vi "ConfigureDlg.vi"(8 "error in (no error)":errorcluster, 11 "NiPxi6682 in":refnum<class "NiPxi6682.lvclass">) -> (0 "error out":errorcluster, 2 "Changed?":bool, 3 "NiPxi6682 out":refnum<class "NiPxi6682.lvclass">)   [LabVIEW 2014, in "SyncPlugins.lvlib" / "NiPxi6682.lvclass"]
uses:
  NiPxi6682.lvclass
  NiPxi6682.lvclass/NiPxi6682.ctl
  <userlib>/NIST/BaseClasses/BasePlugin_class/BasePlugin.lvclass/BasePlugin.ctl
  Accessors/Write 1PPS.vi
  Accessors/Write PgmPPS.vi
  Accessors/Write PgmPPSFreq.vi
  Accessors/Write DdsFreq.vi
  <userlib>/NIST/BaseClasses/BasePlugin_class/Accessors/Read PluginIniFilePath.vi
  Accessors/Read 1PPS.vi
  Accessors/Read PgmPPS.vi
  Accessors/Read PgmPPSFreq.vi
  Accessors/Read DdsFreq.vi
  <vilib>/Utility/config.llb/NI_LVConfig.lvlib
panel:
  in  "DDSFreq":dbl=100.0 caption="Backplane Clock Freq" format="%#.2p"
  in  "btnCancel":bool
  in  "btnDone":bool
  in  "Programmable Out Port":string
  in  "PgmPPSFreq":dbl=100.0 caption="Programable Out Freq"
  in  "PPS Out Port":string
  in  "Timing Card Handle":string
  in  "Clock Card Handle":string
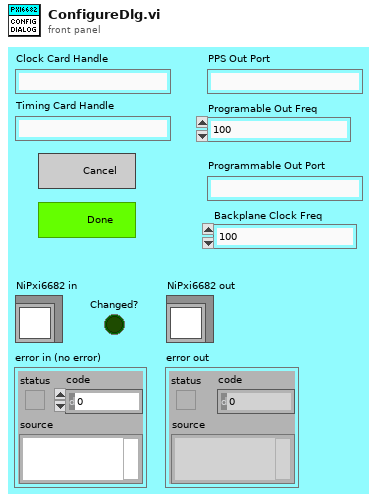
[diagram p1: front panel]
types:
  T1 = enum32{"Invalid", "Default", "Floating", "Floating/Auto-Hide", "Modal"}
  T2 = typedef "NI_LVConfig.lvlib/Config Data RefNum.ctl" = refnum<k1>
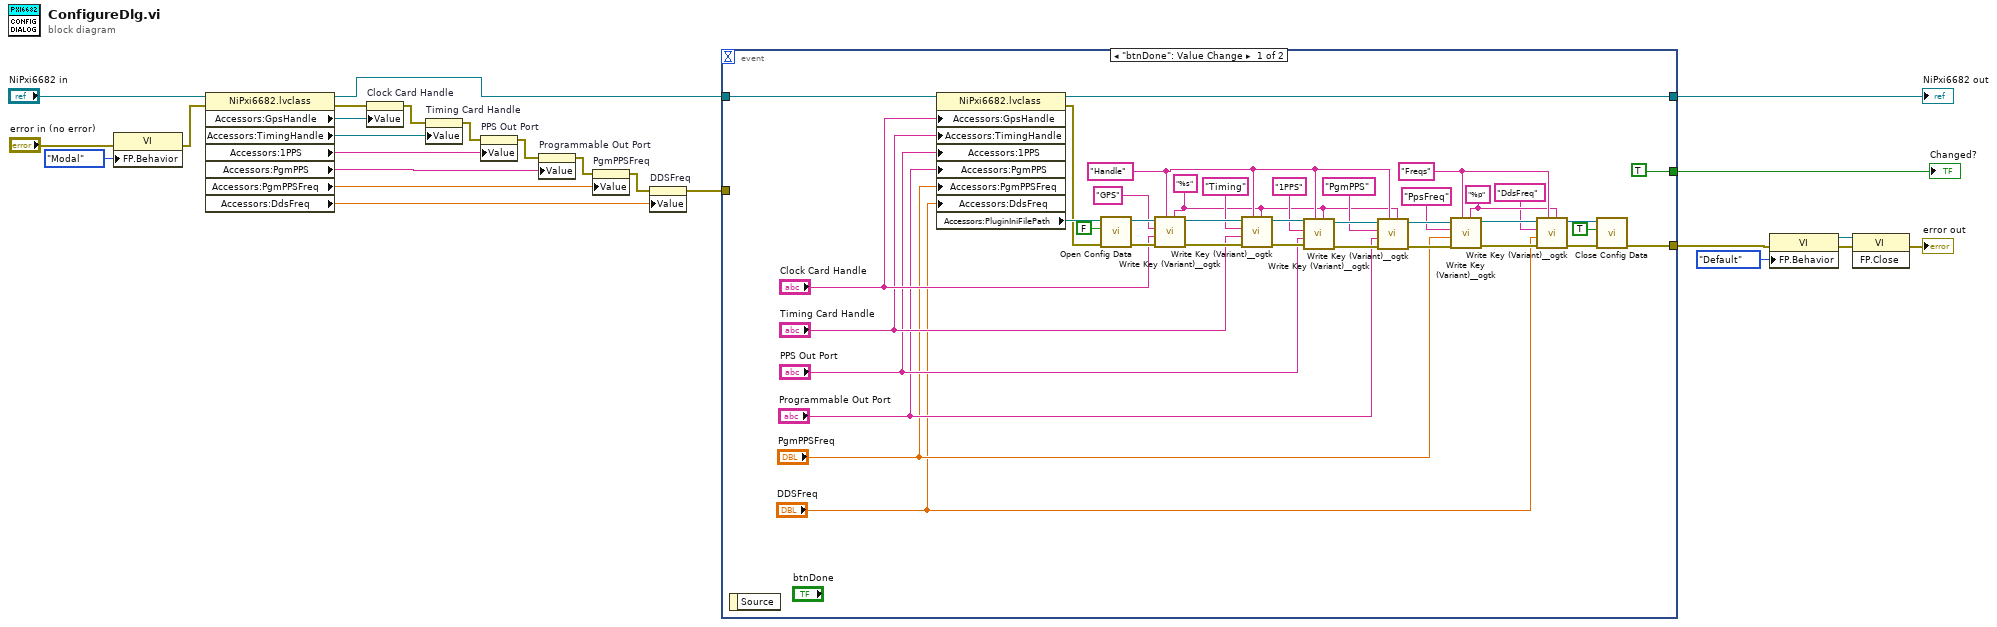
[diagram p0: block diagram]
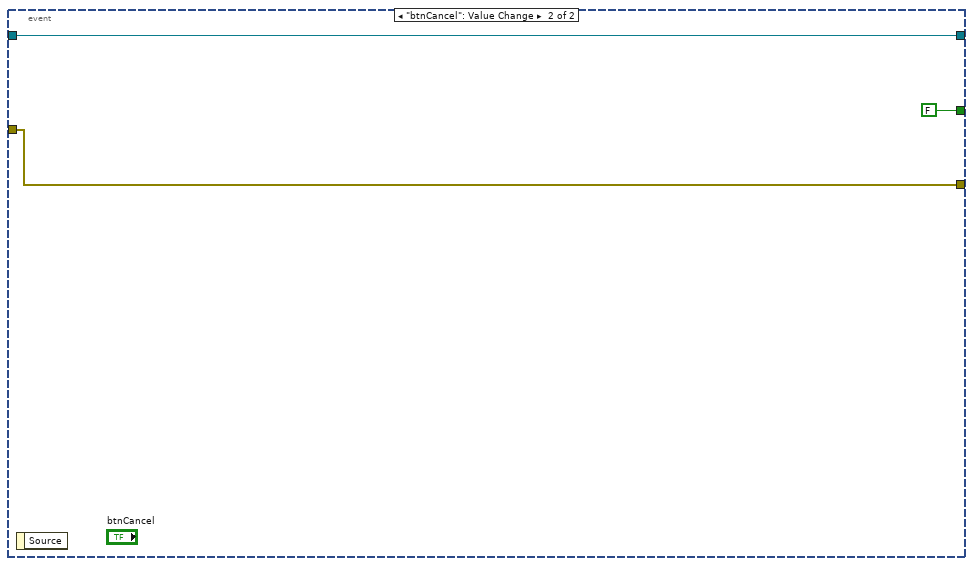
[diagram p2: hidden frame]
diagram:
  n1 = property class="VI"(error in="error in (no error)", "FP.Behavior"=T1."Modal" ("Front Panel Window:Behavior")) -> (error out=w22:errorcluster)  [unwired: 1 in, 1 out]
  n2 = property class="NiPxi6682.lvclass"(reference="NiPxi6682 in", error in=w22) -> (reference out=w7:refnum<class "NiPxi6682.lvclass">, error out=w17:errorcluster, "Accessors:GpsHandle"=w16:refnum<k15>, "Accessors:TimingHandle"=w15:refnum<k15>, "Accessors:1PPS"=w13:tag, "Accessors:PgmPPS"=w10:tag, "Accessors:PgmPPSFreq"=w9:dbl, "Accessors:DdsFreq"=w6:dbl)
  n3 = property on="Clock Card Handle" class="Str"(error in=w17, "Value"=w16) -> (error out=w14:errorcluster)  [unwired: 1 in, 1 out]
  n4 = property on="Timing Card Handle" class="Str"(error in=w14, "Value"=w15) -> (error out=w12:errorcluster)  [unwired: 1 in, 1 out]
  n5 = property on="PPS Out Port" class="Str"(error in=w12, "Value"=w13) -> (error out=w11:errorcluster)  [unwired: 1 in, 1 out]
  n6 = property on="Programmable Out Port" class="Str"(error in=w11, "Value"=w10) -> (error out=w8:errorcluster)  [unwired: 1 in, 1 out]
  n7 = property on="PgmPPSFreq" class="DigNum (strict)"(error in=w8, "Value"=w9) -> (error out=w5:errorcluster)  [unwired: 1 in, 1 out]
  n8 = property on="DDSFreq" class="DigNum (strict)"(error in=w5, "Value"=w6) -> (error out=w4:errorcluster)  [unwired: 1 in, 1 out]
  n9 = event shown="[0] \"btnDone\": Value Change" {
    selector: _ -> [_ _]
    dyn-events: _ -> [_ _]
    timeout: _ -> [_ _]
    tunnel: w7 -> [w63 w65]
    tunnel: w4 -> [_ w66]
    tunnel: [w28 w66] -> w3
    tunnel: [w27 w65] -> w2
    tunnel: [TRUE FALSE] -> w1
    event "btnDone": Value Change {
      w36 = "%p" ("float number format")
      w37 = "Freqs"
      w43 = "%s" ("float number format")
      w44 = "Handle"
      n10 = event-data() -> ()  [unwired: 1 in, 1 out]
      n11 = property class="NiPxi6682.lvclass"(reference=w63, "Accessors:GpsHandle"="Clock Card Handle", "Accessors:TimingHandle"="Timing Card Handle", "Accessors:1PPS"="PPS Out Port", "Accessors:PgmPPS"="Programmable Out Port", "Accessors:PgmPPSFreq"="PgmPPSFreq", "Accessors:DdsFreq"="DDSFreq") -> (reference out=w27:refnum<class "NiPxi6682.lvclass">, error out=w61:errorcluster, "Accessors:PluginIniFilePath"=w62:path)  [unwired: 1 in]
      n12 = call <vilib>:"Open Config Data.vi"("error in (no error)"=w61, "create file if necessary (T)"=FALSE, "configuration file path"=w62) -> ("error out"=w59:errorcluster, "refnum"=w58:T2)  [unwired: 6 in, 1 out]
      n13 = call <userlib>:"Write Key (Variant)__ogtk.vi"("float number format"=w43, "section"=w44, "error in (no error)"=w59, "key-value"="Clock Card Handle", "key (optional)"="GPS", "refnum"=w58) -> ("error out"=w56:errorcluster, "refnum out"=w55:T2)  [unwired: 4 in]
      n14 = call <userlib>:"Write Key (Variant)__ogtk.vi"("float number format"=w43, "section"=w44, "error in (no error)"=w56, "key-value"="Timing Card Handle", "key (optional)"="Timing", "refnum"=w55) -> ("error out"=w51:errorcluster, "refnum out"=w50:T2)  [unwired: 4 in]
      n15 = call <userlib>:"Write Key (Variant)__ogtk.vi"("float number format"=w43, "section"=w44, "error in (no error)"=w51, "key-value"="PPS Out Port", "key (optional)"="1PPS", "refnum"=w50) -> ("error out"=w47:errorcluster, "refnum out"=w46:T2)  [unwired: 4 in]
      n16 = call <userlib>:"Write Key (Variant)__ogtk.vi"("float number format"=w43, "section"=w44, "error in (no error)"=w47, "key-value"="Programmable Out Port", "key (optional)"="PgmPPS", "refnum"=w46) -> ("error out"=w41:errorcluster, "refnum out"=w40:T2)  [unwired: 4 in]
      n17 = call <userlib>:"Write Key (Variant)__ogtk.vi"("float number format"=w36, "section"=w37, "error in (no error)"=w41, "key-value"="PgmPPSFreq", "key (optional)"="PpsFreq", "refnum"=w40) -> ("error out"=w39:errorcluster, "refnum out"=w38:T2)  [unwired: 4 in]
      n18 = call <userlib>:"Write Key (Variant)__ogtk.vi"("float number format"=w36, "section"=w37, "error in (no error)"=w39, "key-value"="DDSFreq", "key (optional)"="DdsFreq", "refnum"=w38) -> ("error out"=w31:errorcluster, "refnum out"=w30:T2)  [unwired: 4 in]
      n19 = call <vilib>:"Close Config Data.vi"("error in (no error)"=w31, "write file if changed (T)"=TRUE, "refnum"=w30) -> ("error out"=w28:errorcluster)  [unwired: 7 in, 1 out]
    }
    event "btnCancel": Value Change {
      n20 = event-data() -> ()  [unwired: 1 in, 1 out]
    }
  }
  "NiPxi6682 out" <- w2
  "Changed?" <- w1
  n21 = property class="VI"(error in=w3, "FP.Behavior"=T1."Default" ("Front Panel Window:Behavior")) -> (reference out=w21:refnum<vi>, error out=w20:errorcluster)  [unwired: 1 in]
  n22 = invoke class="VI" method="FP.Close"(reference=w21, error in=w20) -> (error out=→"error out":errorcluster)  [unwired: 1 in, 2 out]
